vi "Analysator initialisieren.vi"(7 "byName":bool, 8 "error in (no error)":errorcluster caption="Fehler (Eingang, kein Fehler)", 11 "Referenz Analysator":refnum<vi>) -> (0 "error out":errorcluster caption="Fehler (Ausgang)", 3 "Referenz Analysator out":refnum<vi>)   [LabVIEW 2020, in "System Einstellungen V2.lvlib"]
uses:
  System Einstellungen V2.lvlib
  Aktion FGV SystemEinstellungenV2.ctl
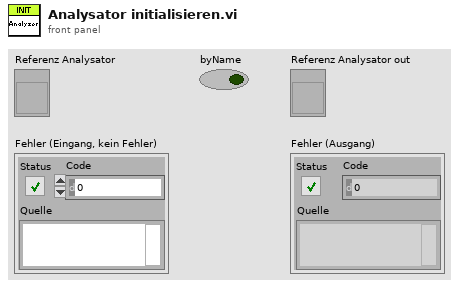
[diagram p1: front panel]
types:
  T1 = typedef "System Einstellungen V2.lvlib/Aktion FGV SystemEinstellungenV2.ctl" = enum16{"lesen", "Analysatoren schreiben", "Analysator ändern", "Analysatoren löschen", "laden", "speichern", "Untertitel", "Analysatoren", "Neue Analysatoren", "Gasteiler schreiben", "Gasteiler ändern", "Gasteiler löschen", "Gasteiler", "Gasteiler exportieren", "Gasteiler importieren"}
  T2 = typedef "System Einstellungen V2.lvlib/AnalysatorDefinition.ctl" = cluster{"Analysator":string, "Name für Protokoll":string, "Type":string, "Seriennummer":string}
  T3 = typedef "LVComboBoxStrsAndValuesArrayTypeDef.ctl" = cluster{"String":string, "Value":string}[]
  T4 = cluster{"AnalysatorDefinitionListe":T2[], "AnalysatorDefinitionTextListe":string[][], "Analysatoren Strings And Values[]":T3}
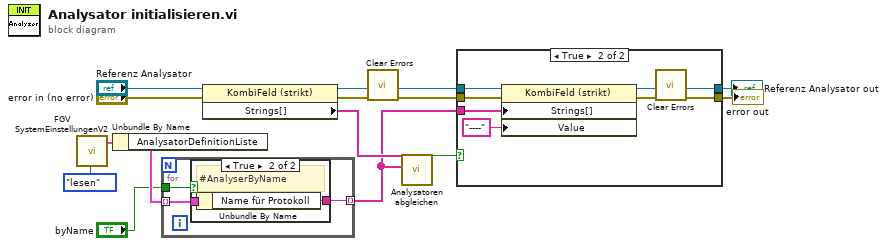
[diagram p0: block diagram]
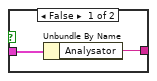
[diagram p2: hidden frame]
diagram:
  n1 = call "FGV SystemEinstellungenV2.vi"("Aktion"=Aktion_FGV_SystemEinstellungenV2."lesen") -> ("Analysatoren"=w7:T4)  [unwired: 5 in, 5 out]
  n2 = Unbundle By Name(w7) -> ("AnalysatorDefinitionListe"=w8:T2[])
  n3 = for {
    tunnel: w8 -> [w17] mode=indexing
    tunnel: [w16] -> w6 mode=indexing
    tunnel: "byName" -> [w15]
    n4 = case shown="True" w15 {
      tunnel: w17 -> [w19 w21]
      tunnel: [w18 w20] -> w16
      frame False {
        n5 = Unbundle By Name(w19) -> ("Analysator"=w18:string)
      }
      frame True {
        # "#AnalyserByName"
        n6 = Unbundle By Name(w21) -> ("Name für Protokoll"=w20:string)
      }
    }
  }
  n7 = property class="KombiFeld (strikt)"(reference="Referenz Analysator", error in="error in (no error)") -> (reference out=w11:refnum<vi>, error out=w14:errorcluster, "Strings[]"=w12:string[])
  n8 = call <vilib>:"Clear Errors.vi"("error in (no error)"=w14) -> ("error out"=w4:errorcluster)  [unwired: 5 in, 1 out]
  n9 = call "Analysatoren abgleichen.vi"("Analysatorliste"=w6, "Analysatoren"=w12) -> ("x != y?"=w13:bool)  [unwired: 9 in]
  n10 = case shown="True" w13 {
    tunnel: w11 -> [w22 w28]
    tunnel: w6 -> [_ w29]
    tunnel: w4 -> [w23 w26]
    tunnel: [w23 w25] -> w3
    tunnel: [w22 w24] -> w1
    frame False {
    }
    frame True {
      n11 = property class="KombiFeld (strikt)"(reference=w28, error in=w26, "Strings[]"=w29, "Value"="----") -> (reference out=w24:refnum<vi>, error out=w30:errorcluster)
      n12 = call <vilib>:"Clear Errors.vi"("error in (no error)"=w30) -> ("error out"=w25:errorcluster)  [unwired: 5 in, 1 out]
    }
  }
  "error out" <- w3
  "Referenz Analysator out" <- w1
